vi "read.vi"(0 "handle":i32, 5 "Reset M1":bool, 7 "Reset M2":bool, 9 "Reset M3":bool, 11 "Reset Encoders":bool) -> (8 "M1 pos":dbl, 10 "M2 pos":dbl, 15 "M3 pos":dbl)   [LabVIEW 2012]
uses:
  MicroDrive.dll
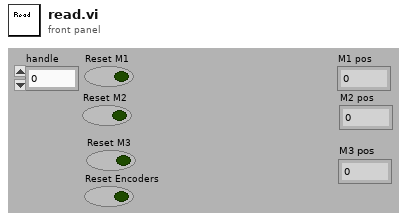
[diagram p1: front panel]
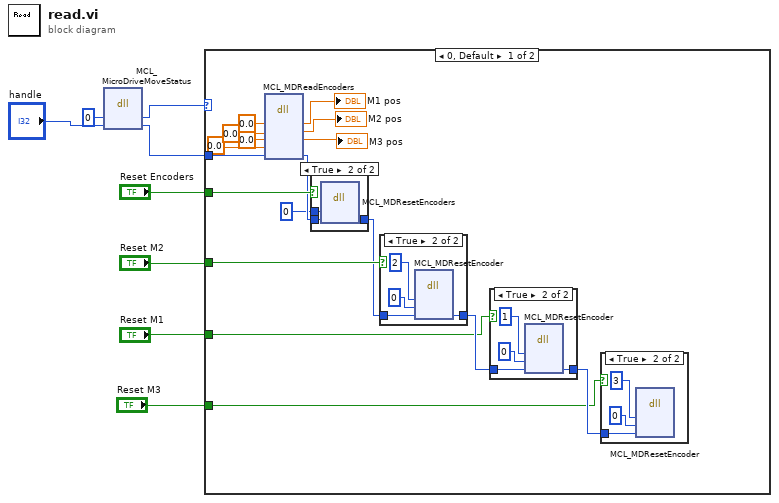
[diagram p0: block diagram]
diagram:
  n1 = dll-call lib="C:/Users/Labview/Desktop/SRR/MicroDrive_x64/Labview Examples/MicroDrive.dll" fn="MCL_MicroDriveMoveStatus"("isMoving"=0, "handle"="handle") -> ("isMoving"=w6:i32, "handle"=w5:i32)  [unwired: 3 in, 3 out]
  n2 = case shown="0, Default" w6 {
    tunnel: w5 -> [w23 _]
    tunnel: "Reset Encoders" -> [w22 _]
    tunnel: "Reset M2" -> [w21 _]
    tunnel: "Reset M1" -> [w10 _]
    tunnel: "Reset M3" -> [w9 _]
    frame 0, Default {
      n3 = dll-call lib="C:/Users/Labview/Desktop/SRR/MicroDrive_x64/Labview Examples/MicroDrive.dll" fn="MCL_MDReadEncoders"("e1"=0.0 ("x enc"), "e2"=0.0 ("y enc"), "e3"=0.0 ("z enc"), "e4"=0.0 ("y enc"), "handle"=w23) -> ("e1"=→"M1 pos":dbl, "e2"=→"M2 pos":dbl, "e3"=→"M3 pos":dbl, "handle"=w20:i32)  [unwired: 3 in, 4 out]
      n4 = case shown="True" w22 {
        tunnel: w20 -> [w39 w42]
        tunnel: [w39 w41] -> w19
        tunnel: u16 0 ("status") -> [_ w40]
        frame False {
        }
        frame True {
          n5 = dll-call lib="C:/Users/Labview/Desktop/SRR/MicroDrive_x64/Labview Examples/MicroDrive.dll" fn="MCL_MDResetEncoders"("status"=w40, "handle"=w42) -> ("handle"=w41:i32)  [unwired: 3 in, 4 out]
        }
      }
      n6 = case shown="True" w21 {
        tunnel: w19 -> [w34 w38]
        tunnel: [w34 w35] -> w12
        frame False {
        }
        frame True {
          n7 = dll-call lib="C:/Users/Labview/Desktop/SRR/MicroDrive_x64/Labview Examples/MicroDrive.dll" fn="MCL_MDResetEncoder"("axis"=u32 2 ("status"), "status"=u16 0, "handle"=w38) -> ("handle"=w35:i32)  [unwired: 3 in, 5 out]
        }
      }
      n8 = case shown="True" w10 {
        tunnel: w12 -> [w29 w33]
        tunnel: [w29 w30] -> w11
        frame False {
        }
        frame True {
          n9 = dll-call lib="C:/Users/Labview/Desktop/SRR/MicroDrive_x64/Labview Examples/MicroDrive.dll" fn="MCL_MDResetEncoder"("axis"=u32 1 ("status"), "status"=u16 0, "handle"=w33) -> ("handle"=w30:i32)  [unwired: 3 in, 5 out]
        }
      }
      n10 = case shown="True" w9 {
        tunnel: w11 -> [_ w28]
        frame False {
        }
        frame True {
          n11 = dll-call lib="C:/Users/Labview/Desktop/SRR/MicroDrive_x64/Labview Examples/MicroDrive.dll" fn="MCL_MDResetEncoder"("axis"=u32 3 ("status"), "status"=u16 0, "handle"=w28) -> ()  [unwired: 4 in, 5 out]
        }
      }
    }
    frame 1 {
    }
  }
